vi "genIOL_Injection.vi"(0 "Iris path":path=path "D:/IRISSoft LV2016 beta/Host Demo/ThorlabsData/Eye1/VSCAN_0002.raw", 1 "PC path":path=path "D:/IRISSoft LV2016 beta/Host Demo/ThorlabsData/Eye1/VSCAN_0003.raw", 2 "endPt":dbl[](array[numeric]), 3 "OCT offset":dbl=13.0) -> ()   [LabVIEW 2016]
uses:
  <vilib>/Math Plots/3D Math Plots/3D Scatter/3D Scatter XCtrl/3D Scatter.xctl
  <vilib>/Math Plots/3D Math Plots/3D Scatter/3D Scatter Datatype/Public/Plot Helper (Vector).vi
  <vilib>/Analysis/NI_AALBase.lvlib
  <vilib>/Analysis/1siggen.llb/Ramp Pattern by Samples.vi
  <vilib>/gmath/NI_Gmath.lvlib
  Subsystems/Global Variables.vi
  <vilib>/Math Plots/3D Math Plots/3D Scatter/3D Scatter Datatype/3D Scatter Datatype.lvclass
panel:
  out "Incision point":dbl[](array[numeric])
  out "Implement Injection Plot":refnum<class "3D Plot Datatype.lvclass">[](xcontrol)
  out "Implement joint angles":dbl[][](graph)
  out "min dist":dbl
  out "Actual Injection Plot":refnum<class "3D Plot Datatype.lvclass">[](xcontrol)
  out "End manual joint":dbl[](array[numeric])
  out "Start manual joint":dbl[](array[numeric])
  out "Planed joint angles":dbl[][](graph)
  out "Whole joint angles":dbl[][](graph)
  out "traj":dbl[][](array[numeric])
  out "max dist":dbl
  out "Offset":dbl[][](array[numeric])
  out "Incision point index":dbl
  out "Planed Injection Plot":refnum<class "3D Plot Datatype.lvclass">[](xcontrol)
  out "current loop #":dbl
  out "x coordinates size 3":dbl
  out "x coordinates size 2":dbl
  out "x coordinates size":dbl
  out "x coordinates":dbl[](array[numeric])
  out "z coordinates":dbl[](array[numeric]) format="%#_13g"
  out "y coordinates":dbl[](array[numeric]) format="%#_13g"
  out "x coodi 2nd":dbl[](array[numeric]) format="%#_13g"
  in  "Total Time":dbl=60.0
  in  "Arm ID Ind":i32
  in  "Tip out Posit":dbl[](array[numeric])=[0.0, 0.0, 0.0] caption="Position [mm]" format="%#.3f"
  in  "Cycle Time [sec]":dbl[](array[numeric])=[60.0, 90.0, 120.0]
  out "zVisTraj":dbl[](array[numeric]) format="%_6g"
  out "yVisTraj":dbl[](array[numeric]) format="%_6g"
  out "xVisTraj":dbl[](array[numeric]) format="%_6g"
  in  "Sampling Rate [Hz]":i32=1000
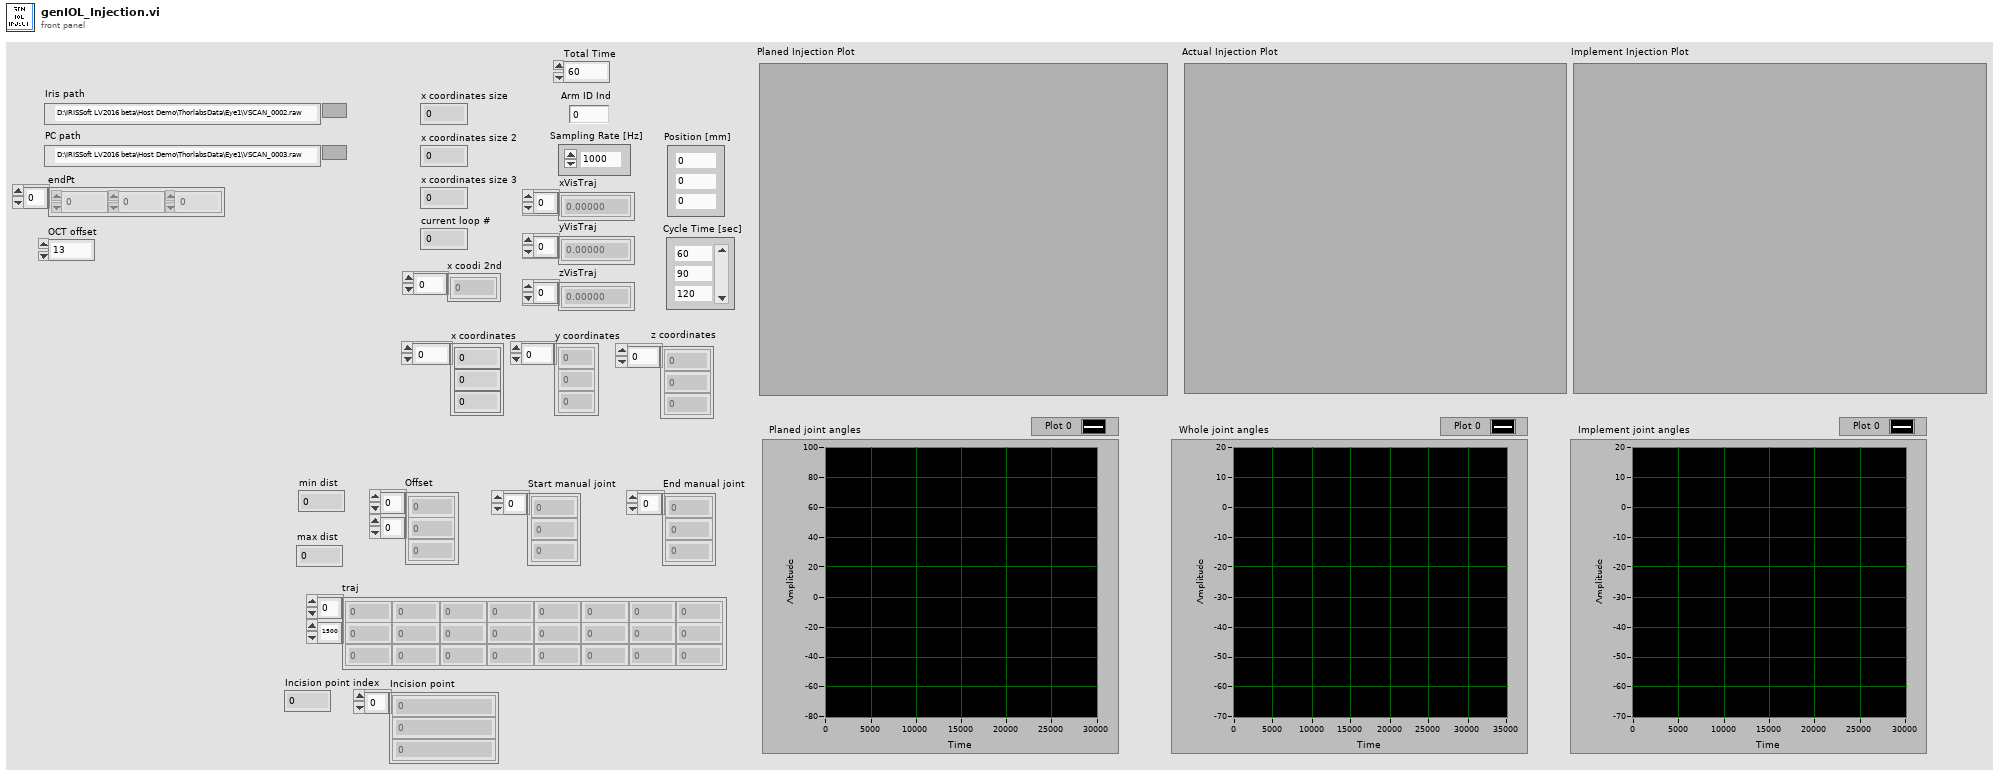
[diagram p1: front panel]
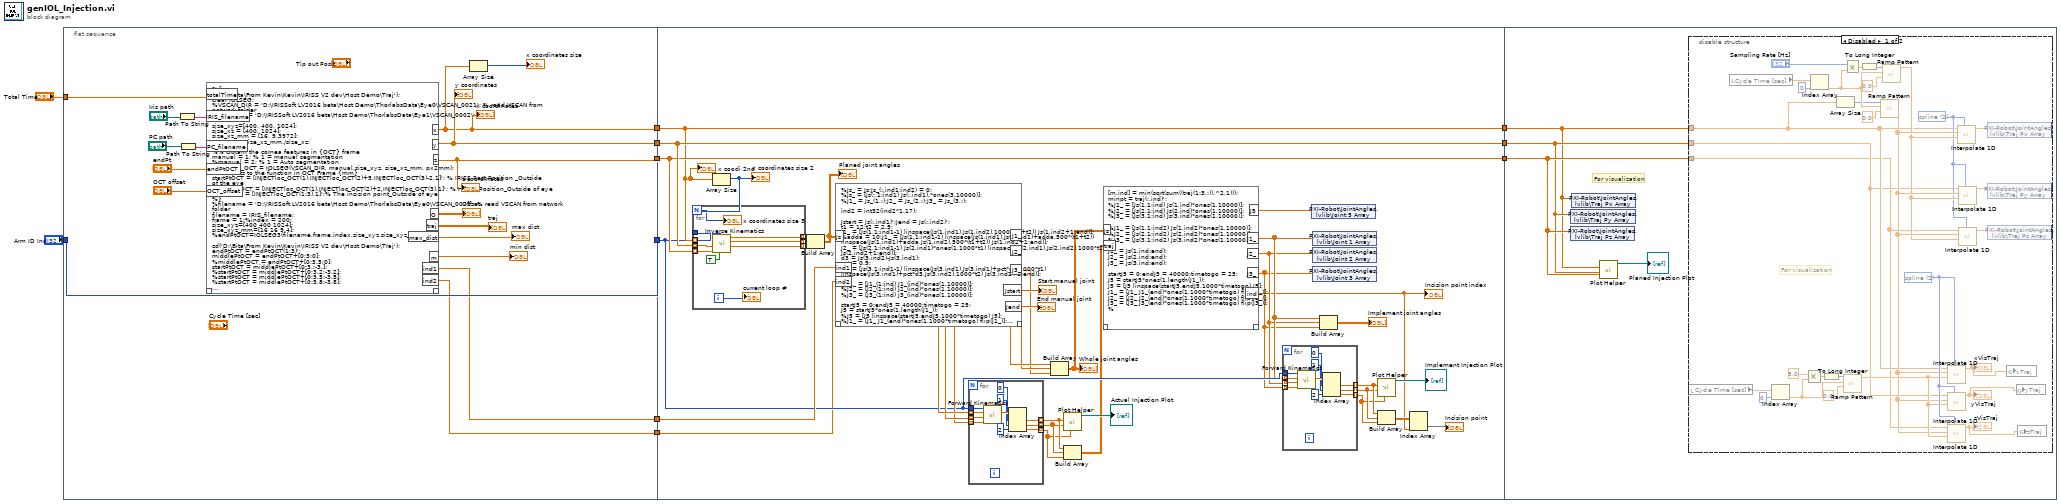
[diagram p0: block diagram]
diagram:
  n1 = flat-sequence {
    tunnel: "Arm ID Ind" -> [w29]
    tunnel: [w29] -> w10
    tunnel: [w25] -> w6
    tunnel: [w27] -> w5
    tunnel: [w26] -> w4
    tunnel: "Total Time" -> [w28]
    tunnel: [w20] -> w2
    tunnel: [w19] -> w1
    tunnel: w10 -> [w40]
    tunnel: [w61] -> w9
    tunnel: [w63] -> w8
    tunnel: [w62] -> w7
    tunnel: w6 -> [w61]
    tunnel: w5 -> [w63]
    tunnel: w4 -> [w62]
    tunnel: w2 -> [w56]
    tunnel: w1 -> [w30]
    tunnel: w9 -> [w96]
    tunnel: w8 -> [w97]
    tunnel: w7 -> [w98]
    frame #0 {
      n2 = Path To String(path="Iris path") -> (string=w16:string)
      n3 = Path To String(path="PC path") -> (string=w17:string)
      n4 = script code="%{\ncd('D:\\Bita\\From Kevin\\Kevin\\IRISS V2 dev\\Host Demo\\Traj');\nclear IOLSEG;\n%VSCAN_DIR = 'D:\\IRISSoft LV2016 beta\\Host Demo\\ThorlabsData\\Eye0\\VSCAN_0021'; % read VSCAN from network folder \nVSCAN_DIR = 'D:\\IRISSoft LV2016 beta\\Host Demo\\ThorlabsData\\Eye1\\VSCAN_0002';\n\nsize_xyz=[400, 400, 1024];\nsize_xz = [400, 1024]; \nsize_xz_mm = [16, 9.3972]; \npx2mm = size_xz_mm./size_xz; \n    \n%% Obtain the cornea features in {OCT} frame\nmanual = 1; % 1 = manual segmentation\n%manual = 2; % 1 = Auto segmentation\nINJECTloc_OCT = IOLSEG(VSCAN_DIR, manual,size_xyz, size_xz_mm, px2mm);\n%% inputs to the function in OCT Frame {mm}\nstartPtOCT = [INJECTloc_OCT(1),INJECTloc_OCT(2)+5,INJECTloc_OCT(3)-2,1]'; % IRISS Rest Position _Outside of the eye\nmiddlePtOCT = [INJECTloc_OCT(1),INJECTloc_OCT(2)+2,INJECTloc_OCT(3),1]'; % Home Position_Outside of eye\nendPtOCT = [INJECTloc_OCT(1:3),1]';% The incision point_Outside of eye\n%}\n%filename = 'D:\\IRISSoft LV2016 beta\\Host Demo\\ThorlabsData\\Eye0\\VSCAN_0021'; % read VSCAN from network folder \nfilename = IRIS_filename;\nframe = 1;%index = 200;\nsize_xyz=[400 400 1024];\nsize_xyz_mm=[16 16 9.4];\n%endPtOCT=IOLSEG3(filename,frame,index,size_xyz,size_xyz_mm);\n\ncd('D:\\Bita\\From Kevin\\Kevin\\IRISS V2 dev\\Host Demo\\Traj');\nendPtOCT = endPtOCT(1:3)';\nmiddlePtOCT = endPtOCT+[0;3;0];\n%middlePtOCT = endPtOCT+[0;3.5;0];\nstartPtOCT = middlePtOCT+[0;3.;-3.];\n%startPtOCT = middlePtOCT+[0;3.2;-3.2];\n%startPtOCT = middlePtOCT+[0;3.5;-3.5];\n%startPtOCT = middlePtOCT+[0;3.8;-3.8];\n\n%middlePtOCT = endPtOCT+[0;-3;0];\n%startPtOCT = middlePtOCT+[0;-3.8;-3.8];\n\n%IRIS_filename = 'D:\\IRISSoft LV2016 beta\\Host Demo\\ThorlabsData\\Eye0\\VSCAN_0021.raw';\n%PC_filename = 'D:\\IRISSoft LV2016 beta\\Host Demo\\ThorlabsData\\Eye0\\VSCAN_0022.raw';\n%OCT_offset = 7; %OCT_offset = 0;\n%IRIS_filename = 'D:\\IRISSoft LV2016 beta\\Host Demo\\ThorlabsData\\Eye1\\VSCAN_0002.raw';\n%PC_filename = 'D:\\IRISSoft LV2016 beta\\Host Demo\\ThorlabsData\\Eye1\\VSCAN_0003.raw';\n%OCT_offset = 13;\nspeed_scaler = 0.15;\n[tts,traj2,ind1,ind2]=IOL_injection_trajectory(startPtOCT,middlePtOCT,endPtOCT,IRIS_filename,PC_filename,OCT_offset,speed_scaler);\nTOI_file= 'D:\\IRISSoft LV2016 beta\\Host Demo\\TOI_static'\nfid_TOI = fopen(TOI_file,'r');\nTOI=fscanf(fid_TOI,'%f');\nTOI= reshape(TOI, [4 4])';\nfclose(fid_TOI);\n\nmax_dist = max(sqrt(sum(diff(traj2,1,2).^2,1)));\nO = inv(TOI)*[endPtOCT;1];\n%{\ninit_X = 40;init_Y = 55;init_Z = 100;\ntime_to_go = norm(O(1:3))/.5;\nstage_X = linspace(init_X,init_X+O(1),1000*time_to_go);\nstage_Y = linspace(init_Y,init_Y+O(2),1000*time_to_go);\nstage_Z = linspace(init_Z,init_Z+O(3),1000*time_to_go);\n%}\n\nTOI2 = inv(TOI);TOI2(1:3,4) = TOI2(1:3,4)-O(1:3);\ntraj = TOI2*[traj2;ones(1,size(traj2,2))];\n%{\nTOI2_file= 'D:\\IRISSoft LV2016 beta\\Host Demo\\new_TOI.txt'\nfid_TOI2 = fopen(TOI2_file,'r');\nTOI2=fscanf(fid_TOI2,'%f');\nTOI2= reshape(TOI2, [4 4]);\nfclose(fid_TOI2);\ntraj = inv(TOI2)*[traj2;ones(1,size(traj2,2))];\n%}\n\nx = traj(1,:);y = traj(2,:);z = traj(3,:);\n[m,ind] = min(sqrt(sum((traj(1:3,:)).^2,1)));"("totalTime"=w28, "IRIS_filename"=w16, "PC_filename"=w17, "endPtOCT"="endPt", "OCT_offset"="OCT offset") -> ("x"=w25:dbl[], "y"=w27:dbl[], "z"=w26:dbl[], "O"=→"Offset":dbl[][], "max_dist"=→"max dist":dbl, "traj"=→"traj":dbl[][], "ind1"=w20:dbl, "ind2"=w19:dbl, "m"=→"min dist":dbl)  [unwired: 1 in, 1 out]
      "y coordinates" <- w27
      "z coordinates" <- w26
      "x coordinates" <- w25
      n5 = Array Size(array=w25) -> (size(s)=→"x coordinates size":i32)
    }
    frame #1 {
      n6 = Array Size(array=w61) -> (size(s)=w60:i32)
      "x coordinates size 2" <- w60
      n7 = for {
        N: w60 -> [w90]
        tunnel: w40 -> [w91]
        tunnel: w61 -> [w95] mode=indexing
        tunnel: w63 -> [w94] mode=indexing
        tunnel: w62 -> [w93] mode=indexing
        tunnel: [w88] -> w58 mode=indexing
        tunnel: [w87] -> w57 mode=indexing
        tunnel: [w86] -> w59 mode=indexing
        i -> [w89]
        n8 = call "Inverse Kinematics.vi"("isToolTipInsideEye"=TRUE, "armID"=w91, "z"=w93, "y"=w94, "x"=w95) -> ("j3"=w87:dbl, "j2"=w88:dbl, "j1"=w86:dbl)  [unwired: 3 in, 1 out]
        "x coordinates size 3" <- w90
        "current loop #" <- w89
      }
      n9 = Build Array(w59, w58, w57) -> (w55:dbl[][])
      "Planed joint angles" <- w55
      n10 = script code="%Js_ = Js;Js_(:,ind1:ind2) = 0;\n%Js_ = [Js(:,1:ind1) Js(:,ind1).*ones(3,10000)];\n%J1_ = Js_(1,:);J2_ = Js_(2,:);J3_ = Js_(3,:);\n\nind2 = int32(ind2*1.17);\n\nJstart = Js(:,ind1)';Jend = Js(:,ind2)';\nt1 = 12;t2 = 2.5;\nJ1_ = [Js(1,1:ind1-1) linspace(Js(1,ind1),Js(1,ind2),1000*(t1+t2)) Js(1,ind2+1:end)];\n%adda = 10;J1_ = [Js(1,1:ind1-1) linspace(Js(1,ind1),Js(1,ind1)+adda,500*(t1+t2)) linspace(Js(1,ind1)+adda,Js(1,ind2),500*(t1+t2)) Js(1,ind2+1:end)];\nJ2_ = [Js(2,1:ind1-1) Js(2,ind1)*ones(1,1000*t1) linspace(Js(2,ind1),Js(2,ind2),1000*t2) Js(2,ind2+1:end)];\nd3 = Js(3,ind2)-Js(3,ind1);\npct = 0.9;\nJ3_ = [Js(3,1:ind1-1) linspace(Js(3,ind1),Js(3,ind1)+pct*d3,1000*t1) linspace(Js(3,ind1)+pct*d3,Js(3,ind2),1000*t2) Js(3,ind2+1:end)];\n\n%J1_ = [J1_(1:ind) J1_(ind)*ones(1,10000)];\n%J2_ = [J2_(1:ind) J2_(ind)*ones(1,10000)];\n%J3_ = [J3_(1:ind) J3_(ind)*ones(1,10000)];\n\nstartJ5 = 0;endJ5 = 40000;timetogo = 25;\nJ5 = startJ5*ones(1,length(J1_));\n%J5 = [J5 linspace(startJ5,endJ5,1000*timetogo) J5];\n%J1_ = [J1_ J1_(end)*ones(1,1000*timetogo) flip(J1_)];\n%J2_ = [J2_ J2_(end)*ones(1,1000*timetogo) flip(J2_)];\n%J3_ = [J3_ J3_(end)*ones(1,1000*timetogo) flip(J3_)];"("Js"=w55, "ind1"=w56, "ind2"=w30) -> ("J1_"=w52:dbl[], "J2_"=w51:dbl[], "J3_"=w50:dbl[], "Jstart"=→"Start manual joint":dbl[], "Jend"=→"End manual joint":dbl[])  [unwired: 1 in, 1 out]
      n11 = for {
        tunnel: w40 -> [w85]
        tunnel: w52 -> [w84] mode=indexing
        tunnel: w51 -> [w83] mode=indexing
        tunnel: w50 -> [w82] mode=indexing
        tunnel: [w77] -> w48 mode=indexing
        tunnel: [w76] -> w47 mode=indexing
        tunnel: [w75] -> w46 mode=indexing
        n12 = call "Forward Kinematics.vi"("j3"=w82, "j2"=w83, "j1"=w84, "armID"=w85) -> ("XYZ Out Array"=w81:dbl[])  [unwired: 7 in]
        n13 = Index Array(array=w81, index #1=0 ("index"), index #2=1 ("index"), index #3=2 ("index")) -> (element #1=w77:dbl, element #2=w76:dbl, element #3=w75:dbl)
      }
      n14 = Build Array(w52, w51, w50) -> (w39:dbl[][])
      "Whole joint angles" <- w39
      n15 = call-poly <vilib>:"Plot Helper.vi"("z vector"=w46, "y vector"=w47, "x vector"=w48) -> ("3D Plot lvclass Array out"=→"Actual Injection Plot":refnum<class "3D Plot Datatype.lvclass">[])  [unwired: 3 in, 5 out]
      n16 = Build Array(w48, w47, w46) -> (w34:dbl[][])
      n17 = script code="[m,ind] = min(sqrt(sum((traj(1:3,:)).^2,1)));\nminpt = traj(:,ind)';\n%J1_ = [Js(1,1:ind) Js(1,ind)*ones(1,10000)];\n%J2_ = [Js(2,1:ind) Js(2,ind)*ones(1,10000)];\n%J3_ = [Js(3,1:ind) Js(3,ind)*ones(1,10000)];\n\n%J1_ = [Js(1,1:ind2) Js(1,ind2)*ones(1,10000)];\n%J2_ = [Js(2,1:ind2) Js(2,ind2)*ones(1,10000)];\n%J3_ = [Js(3,1:ind2) Js(3,ind2)*ones(1,10000)];\n%\nJ1_ = Js(1,ind:end);\nJ2_ = Js(2,ind:end);\nJ3_ = Js(3,ind:end);\n\nstartJ5 = 0;endJ5 = 40000;timetogo = 25;\nJ5 = startJ5*ones(1,length(J1_));\nJ5 = [J5 linspace(startJ5,endJ5,1000*timetogo) J5];\nJ1_ = [J1_ J1_(end)*ones(1,1000*timetogo) flip(J1_)];\nJ2_ = [J2_ J2_(end)*ones(1,1000*timetogo) flip(J2_)];\nJ3_ = [J3_ J3_(end)*ones(1,1000*timetogo) flip(J3_)];\n%"("Js"=w39, "traj"=w34) -> ("J1_"=w38:dbl[], "J2_"=w37:dbl[], "J3_"=w36:dbl[], "ind"=w32:dbl, "J5"=w41:dbl[])  [unwired: 1 in, 1 out]
      "Incision point index" <- w32
      n18 = for {
        tunnel: w40 -> [w74]
        tunnel: w38 -> [w73] mode=indexing
        tunnel: w37 -> [w72] mode=indexing
        tunnel: w36 -> [w71] mode=indexing
        tunnel: [w66] -> w44 mode=indexing
        tunnel: [w65] -> w43 mode=indexing
        tunnel: [w64] -> w42 mode=indexing
        n19 = call "Forward Kinematics.vi"("j3"=w71, "j2"=w72, "j1"=w73, "armID"=w74) -> ("XYZ Out Array"=w70:dbl[])  [unwired: 7 in]
        n20 = Index Array(array=w70, index #1=0 ("index"), index #2=1 ("index"), index #3=2 ("index")) -> (element #1=w66:dbl, element #2=w65:dbl, element #3=w64:dbl)
      }
      n21 = shared-variable "PXI-Robot\\JointAngles.lvlib\\Joint 5 Array"(w41) -> ()  [unwired: 1 in, 1 out]
      n22 = shared-variable "PXI-Robot\\JointAngles.lvlib\\Joint 1 Array"(w38) -> ()  [unwired: 1 in, 1 out]
      n23 = shared-variable "PXI-Robot\\JointAngles.lvlib\\Joint 2 Array"(w37) -> ()  [unwired: 1 in, 1 out]
      n24 = shared-variable "PXI-Robot\\JointAngles.lvlib\\Joint 3 Array"(w36) -> ()  [unwired: 1 in, 1 out]
      n25 = Build Array(w38, w37, w36) -> (→"Implement joint angles":dbl[][])
      n26 = call-poly <vilib>:"Plot Helper.vi"("z vector"=w42, "y vector"=w43, "x vector"=w44) -> ("3D Plot lvclass Array out"=→"Implement Injection Plot":refnum<class "3D Plot Datatype.lvclass">[])  [unwired: 3 in, 5 out]
      n27 = Build Array(w44, w43, w42) -> (w33:dbl[][])
      n28 = Index Array(array=w33, index (col)=w32) -> (element=→"Incision point":dbl[])  [unwired: 1 in]
      "x coodi 2nd" <- w61
    }
    frame #2 {
      # "For visualization"
      n29 = shared-variable "PXI-Robot\\JointAngles.lvlib\\Traj Py Array"(w97) -> ()  [unwired: 1 in, 1 out]
      n30 = shared-variable "PXI-Robot\\JointAngles.lvlib\\Traj Pz Array"(w98) -> ()  [unwired: 1 in, 1 out]
      n31 = shared-variable "PXI-Robot\\JointAngles.lvlib\\Traj Px Array"(w96) -> ()  [unwired: 1 in, 1 out]
      n32 = call-poly <vilib>:"Plot Helper.vi"("z vector"=w98, "y vector"=w97, "x vector"=w96) -> ("3D Plot lvclass Array out"=→"Planed Injection Plot":refnum<class "3D Plot Datatype.lvclass">[])  [unwired: 3 in, 5 out]
      n33 = disable-structure shown="Disabled" {
        disable-tunnel: w96 -> [w105 _]
        disable-tunnel: w97 -> [w104 _]
        disable-tunnel: w98 -> [w103 _]
        frame Disabled {
          w117 = 2 items=["nearest", "linear", "spline", "cubic Hermite", "Lagrange"] ("method")
          w106 = 2 items=["nearest", "linear", "spline", "cubic Hermite", "Lagrange"] ("method")
          # "For visualization"
          n34 = local read "Cycle Time [sec]"() -> (w111:dbl[])
          n35 = local read "Cycle Time [sec]"() -> (w129:dbl[])
          n36 = Index Array(array=w111, index=0) -> (element=w112:dbl)
          n37 = Multiply(x=5.0, y=w112) -> (x*y=w114:dbl)
          n38 = Index Array(array=w129, index=0) -> (element=w122:dbl)
          n39 = To Long Integer(number=w114) -> (32bit integer=w115:i32)
          n40 = Array Size(array=w105) -> (size(s)=w121:i32)
          n41 = call-poly <vilib>:"Ramp Pattern.vi"("start"=0.0, "end"=w112, "samples"=w115) -> ("Ramp Pattern"=w109:dbl[])  [unwired: 7 in, 1 out]
          n42 = Multiply(x="Sampling Rate [Hz]", y=w122) -> (x*y=w125:dbl)
          n43 = To Long Integer(number=w125) -> (32bit integer=w126:i32)
          n44 = call-poly <vilib>:"Ramp Pattern.vi"("start"=0.0, "end"=w122, "samples"=w121) -> ("Ramp Pattern"=w108:dbl[])  [unwired: 7 in, 1 out]
          n45 = call-poly <vilib>:"Ramp Pattern.vi"("start"=0.0, "end"=w122, "samples"=w126) -> ("Ramp Pattern"=w107:dbl[])  [unwired: 7 in, 1 out]
          n46 = call <vilib>:"Interpolate 1D.vi"("method"=w117, "xi"=w109, "X"=w108, "Y"=w105) -> ("yi"=w100:dbl[])  [unwired: 5 in, 2 out]
          "xVisTraj" <- w100
          n47 = call <vilib>:"Interpolate 1D.vi"("method"=w117, "xi"=w109, "X"=w108, "Y"=w104) -> ("yi"=w101:dbl[])  [unwired: 5 in, 2 out]
          "yVisTraj" <- w101
          n48 = call <vilib>:"Interpolate 1D.vi"("method"=w117, "xi"=w109, "X"=w108, "Y"=w103) -> ("yi"=w102:dbl[])  [unwired: 5 in, 2 out]
          "zVisTraj" <- w102
          n49 = call <vilib>:"Interpolate 1D.vi"("method"=w106, "xi"=w107, "X"=w108, "Y"=w105) -> ("yi"=w119:dbl[])  [unwired: 5 in, 2 out]
          n50 = call <vilib>:"Interpolate 1D.vi"("method"=w106, "xi"=w107, "X"=w108, "Y"=w104) -> ("yi"=w120:dbl[])  [unwired: 5 in, 2 out]
          n51 = call <vilib>:"Interpolate 1D.vi"("method"=w106, "xi"=w107, "X"=w108, "Y"=w103) -> ("yi"=w118:dbl[])  [unwired: 5 in, 2 out]
          n52 = shared-variable "PXI-Robot\\JointAngles.lvlib\\Traj Px Array"(w119) -> ()  [unwired: 1 in, 1 out]
          n53 = shared-variable "PXI-Robot\\JointAngles.lvlib\\Traj Py Array"(w120) -> ()  [unwired: 1 in, 1 out]
          n54 = shared-variable "PXI-Robot\\JointAngles.lvlib\\Traj Pz Array"(w118) -> ()  [unwired: 1 in, 1 out]
          n55 = global write "Global Variables.vi" "xTraj"(w100) -> ()
          n56 = global write "Global Variables.vi" "yTraj"(w101) -> ()
          n57 = global write "Global Variables.vi" "zTraj"(w102) -> ()
        }
        frame Enabled {
        }
      }
    }
  }
